vi "Calculate_CountToTemp.vi"(11 "CountInput":u16) -> (3 "TempOutput":dbl format="%#_2g")   [LabVIEW 2019]
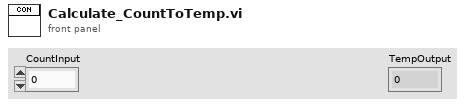
[diagram p1: front panel]
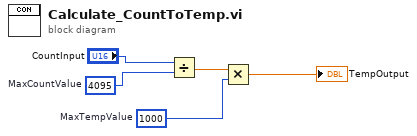
[diagram p0: block diagram]
diagram:
  w4 = u16 4095  # MaxCountValue
  w2 = u16 1000  # MaxTempValue
  n1 = Divide(x="CountInput", y=w4) -> (x/y=w3:dbl)
  n2 = Multiply(x=w3, y=w2) -> (x*y=→"TempOutput":dbl)
